vi "Create LogEngine Obj DVR.vi"(8 "error in (no error)":errorcluster, 11 "LogEngine.lvclass":refnum<class "LogEngine.lvclass">) -> (0 "error out":errorcluster, 3 "LogEngine.lvclass":refnum<class "LogEngine.lvclass">)   [LabVIEW 2022 SP3, in "LogEngine.lvclass"]
doc: "Developed by Kevin Thompson\nkevin@thompsonengineering.net\n\nCopyright 2018-2020\nThompson Engineering, LLC"
uses:
  LogEngine.lvclass
  LogEngine.lvclass/LogEngine.ctl
  Data Types/TD Obj Data_LogEngine.ctl
  Data Types/TD Logger State--enum.ctl
  Data Types/TD Logger State Data--cluster.ctl
  Data Types/TD LogEngine Settings--cluster.ctl
  DataTypes/SessionSettings--cluster.ctl
  Data Types/LogHeaderData--cluster.ctl
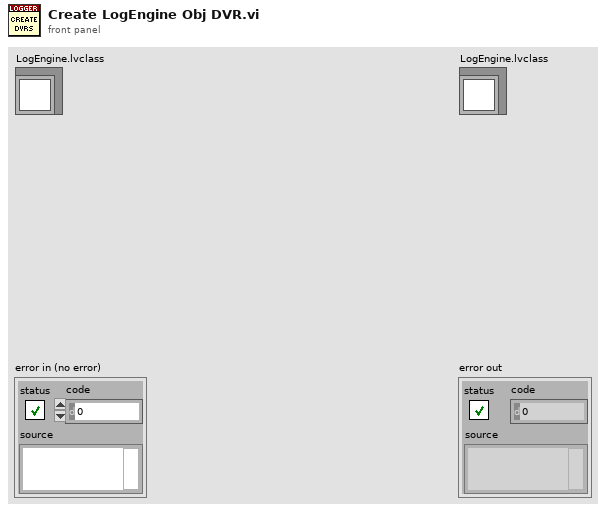
[diagram p1: front panel]
types:
  T1 = typedef "LogEngine.lvclass/TD Obj Data_LogEngine.ctl" = cluster{"LogEngine Settings":T2, "Logger State Data":T3, "tdms fileref":refnum<k34>, "LogHeaderData":T5, "LogHeaderString":string}
  T2 = typedef "LogEngine.lvclass/TD LogEngine Settings--cluster.ctl" = cluster{"placeholder":string, "LogWriteIntv (ms)":u32, "LogFile folder name":string, "TDMS folder name":string}
  T3 = typedef "LogEngine.lvclass/TD Logger State Data--cluster.ctl" = cluster{"Logger State":T4, "TDMS Logging State":T4, "LogFile path":path, "TDMS File path":path, "vData":variant}
  T4 = typedef "LogEngine.lvclass/TD Logger State--enum.ctl" = enum16{"Unknown", "Logging", "NotLogging", "Error"}
  T5 = typedef "LogEngine.lvclass/LogHeaderData--cluster.ctl" = cluster{"SessionSettings":T6, "SequenceFile":string, "Curr_WeldCount":i32, "AI TaskName":string, "SamplingRate":dbl, "SamplesPerAcq":i32}
  T6 = typedef "SessionSettings--cluster.ctl" = cluster{"Job_ID":string, "Operator_ID":string, "Station_ID":string, "Job_Description":string}
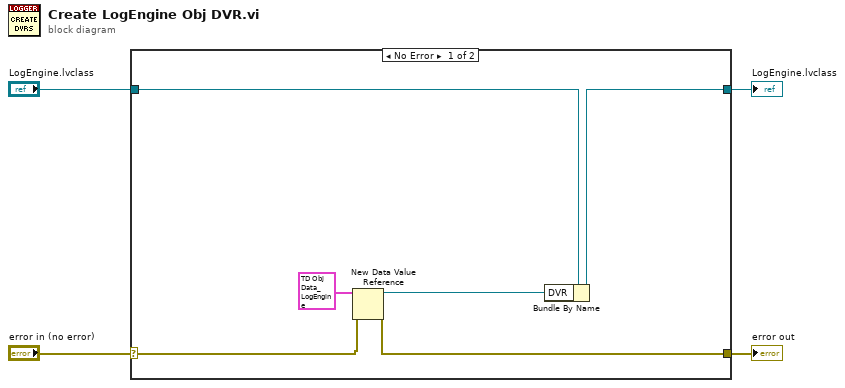
[diagram p0: block diagram]
diagram:
  n1 = case shown="No Error" "error in (no error)" {
    selector: "error in (no error)" -> [w10 w12]
    tunnel: [w9 w12] -> w3
    tunnel: [w7 w11] -> w1
    tunnel: "LogEngine.lvclass" -> [w8 w11]
    frame No Error {
      n2 = New Data Value Reference(data value=T1 {"LogEngine Settings"={"placeholder"="", "LogWriteIntv (ms)"=0, "LogFile folder name"="", "TDMS folder name"=""}, "Logger State Data"={"Logger State"=enum."Unknown", "TDMS Logging State"=enum."Unknown", "LogFile path"=path "", "TDMS File path"=path "", "vData"=variant}, "tdms fileref"=refnum, "LogHeaderData"={"SessionSettings"={"Job_ID"="", "Operator_ID"="", "Station_ID"="", "Job_Description"=""}, "SequenceFile"="", "Curr_WeldCount"=0, "AI TaskName"="", "SamplingRate"=0.0, "SamplesPerAcq"=0}, "LogHeaderString"=""} ("Obj Data"), error in=w10) -> (data value reference=w6:refnum<data-value>, error out=w9:errorcluster)
      n3 = Bundle By Name(cluster=w8, "DVR"=w6) -> (w7:refnum<class "LogEngine.lvclass">)
    }
    frame Error {
    }
  }
  "error out" <- w3
  "LogEngine.lvclass" <- w1
